vi "BumpIntakeLogic.vi"(1 "Initiate":bool) -> (0 "Auto_Bump_Intake":bool)   [LabVIEW 2019]
doc: "This VI performs an automated asymetric \"bump\" sequence on the intake to agitate the ball hopper during shooting."
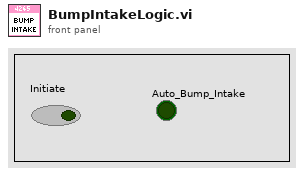
[diagram p1: front panel]
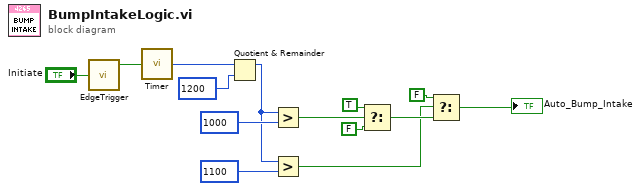
[diagram p0: block diagram]
diagram:
  n1 = call "EdgeTrigger.vi"("Input Signal"="Initiate") -> ("Rising Edge Trigger"=w13:bool)  [unwired: 2 out]
  n2 = call "Timer.vi"("Reset Timer"=w13) -> ("Time (ms)"=w12:u32)
  n3 = Quotient & Remainder(x=w12, y=u32 1200) -> (x-y*floor(x/y)=w3:u32)  [unwired: 1 out]
  n4 = Greater?(x=w3, y=u32 1000) -> (0:w5:bool)
  n5 = Greater?(x=w3, y=u32 1100) -> (0:w2:bool)
  n6 = Select(t=TRUE, s=w5, f=FALSE) -> (s? t:f=w8:bool)
  n7 = Select(t=FALSE, s=w2, f=w8) -> (s? t:f=→"Auto_Bump_Intake":bool)
